vi "GET_Available_TTL_outputs_array.vi"(4 "IO parameters cluster":T1) -> (0 "Disabled items":i32[](array[numeric]), 1 "Available TTL outputs array":cluster{"String":string, "Value":i32}[](array[cluster]))   [LabVIEW 2018, in "Tracker.lvlib"]
uses:
  Tracker.lvlib
  Controls/CTL_IO_params_cluster.ctl
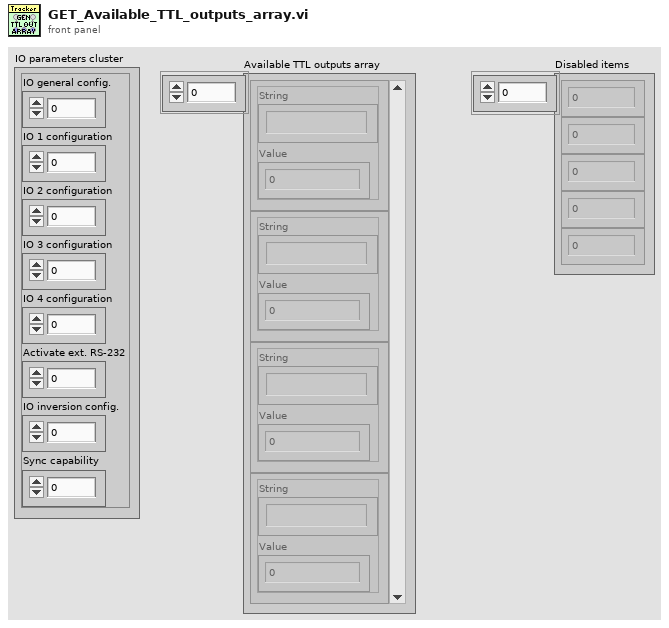
[diagram p1: front panel]
types:
  T1 = typedef "Tracker.lvlib/CTL_IO_params_cluster.ctl" = cluster{"IO general config.":u16, "IO 1 configuration":u16, "IO 2 configuration":u16, "IO 3 configuration":u16, "IO 4 configuration":u16, "Activate ext. RS-232":u16, "IO inversion config.":u16, "Sync capability":u8}
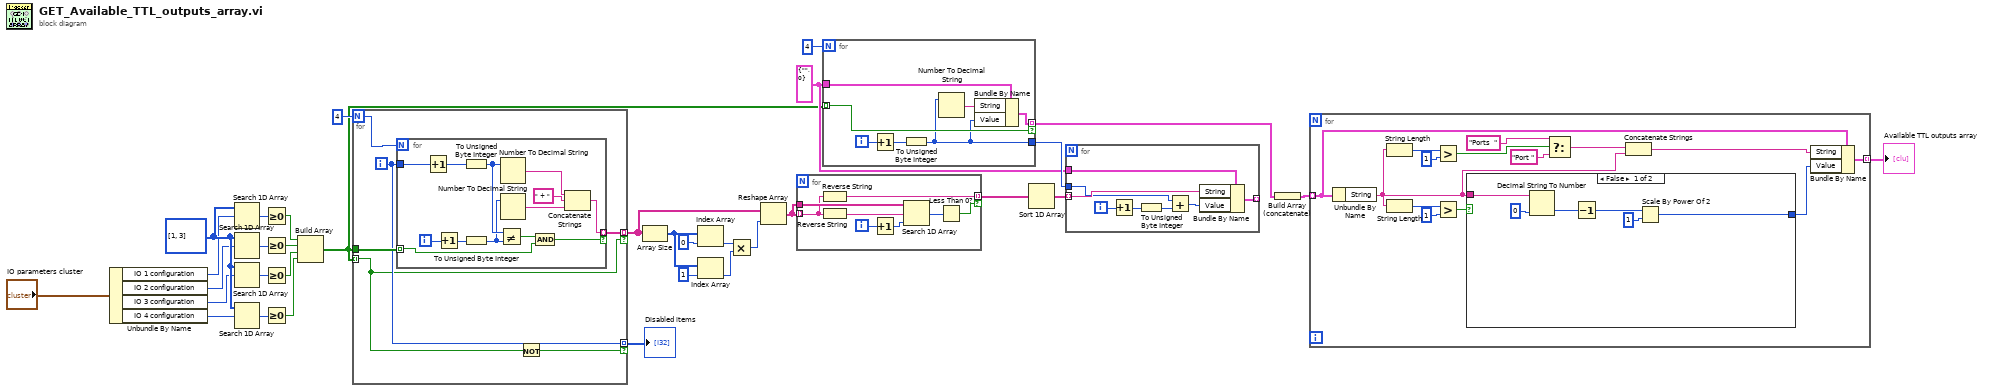
[diagram p0: block diagram]
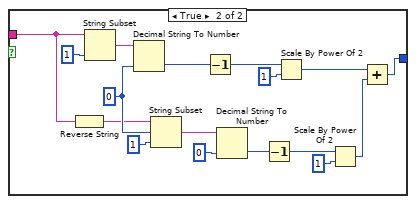
[diagram p2: hidden frame]
diagram:
  w16 = u16[] [1, 3]
  w22 = cluster{"String":string, "Value":u8} {"String"="", "Value"=0} ("Stim. cluster")
  n1 = Unbundle By Name("IO parameters cluster") -> ("IO 1 configuration"=w15:u16, "IO 2 configuration"=w14:u16, "IO 3 configuration"=w13:u16, "IO 4 configuration"=w12:u16)
  n2 = Search 1D Array(1D array=w16, element=w15) -> (index of element=w11:i32)  [unwired: 1 in]
  n3 = Search 1D Array(1D array=w16, element=w14) -> (index of element=w10:i32)  [unwired: 1 in]
  n4 = Search 1D Array(1D array=w16, element=w13) -> (index of element=w9:i32)  [unwired: 1 in]
  n5 = Search 1D Array(1D array=w16, element=w12) -> (index of element=w8:i32)  [unwired: 1 in]
  n6 = Greater Or Equal To 0?(x=w11) -> (x >= 0?=w7:bool)
  n7 = Greater Or Equal To 0?(x=w10) -> (x >= 0?=w6:bool)
  n8 = Greater Or Equal To 0?(x=w9) -> (x >= 0?=w5:bool)
  n9 = Greater Or Equal To 0?(x=w8) -> (x >= 0?=w4:bool)
  n10 = Build Array(w7, w6, w5, w4) -> (w3:bool[])
  n11 = for {
    N: 4 -> [w39]
    tunnel: [w38] -> w31 mode=indexing if=w35
    tunnel: w3 -> [w35] mode=indexing
    tunnel: w3 -> [w37]
    tunnel: [w36] -> w1 mode=indexing if=w34
    i -> [w36]
    n12 = for {
      N: w39 -> [_]
      tunnel: w36 -> [w51]
      tunnel: [w45] -> w38 mode=indexing if=w41
      tunnel: w37 -> [w40] mode=indexing
      i -> [w52]
      n13 = Increment(x=w51) -> (x+1=w50:i32)
      n14 = Increment(x=w52) -> (x+1=w49:i32)
      n15 = To Unsigned Byte Integer(number=w50) -> (unsigned 8bit integer=w44:u8)
      n16 = To Unsigned Byte Integer(number=w49) -> (unsigned 8bit integer=w43:u8)
      n17 = Not Equal?(x=w44, y=w43) -> (x != y?=w42:bool)
      n18 = Number To Decimal String(number=w44) -> (decimal integer string=w48:string)  [unwired: 1 in]
      n19 = Number To Decimal String(number=w43) -> (decimal integer string=w47:string)  [unwired: 1 in]
      n20 = And(x=w42, y=w40) -> (x .and. y?=w41:bool)
      n21 = Concatenate Strings(w48, " + " ("string"), w47) -> (w45:string)
    }
    n22 = Not(x=w35) -> (.not. x?=w34:bool)
  }
  "Disabled items" <- w1
  n23 = Array Size(array=w31) -> (size(s)=w30:i32[])
  n24 = Index Array(array=w30, index=0) -> (element=w27:i32)
  n25 = Index Array(array=w30, index=1) -> (element=w26:i32)
  n26 = Multiply(x=w27, y=w26) -> (x*y=w25:i32)
  n27 = Reshape Array(w31, w25) -> (w24:string[])
  n28 = for {
    tunnel: w24 -> [w58] mode=indexing
    tunnel: [w53] -> w21 mode=indexing if=w56
    tunnel: w24 -> [w60]
    i -> [w55]
    n29 = Reverse String(1:w58) -> (0:w53:string)
    n30 = Reverse String(1:w58) -> (0:w59:string)
    n31 = Increment(x=w55) -> (x+1=w54:i32)
    n32 = Search 1D Array(1D array=w60, element=w59, start index (0)=w54) -> (index of element=w57:i32)
    n33 = Less Than 0?(x=w57) -> (x < 0?=w56:bool)
  }
  n34 = for {
    N: 4 -> [_]
    tunnel: w3 -> [w62] mode=indexing
    tunnel: w22 -> [w65]
    tunnel: [w63] -> w2 mode=indexing if=w62
    tunnel: [w61] -> w23
    i -> [w67]
    n35 = Increment(x=w67) -> (x+1=w66:i32)
    n36 = To Unsigned Byte Integer(number=w66) -> (unsigned 8bit integer=w61:u8)
    n37 = Number To Decimal String(number=w61) -> (decimal integer string=w64:string)  [unwired: 1 in]
    n38 = Bundle By Name(cluster=w65, "String"=w64, "Value"=w61) -> (w63:cluster{"String":string, "Value":u8})
  }
  n39 = Sort 1D Array(array=w21) -> (sorted array=w20:string[])
  n40 = for {
    tunnel: w20 -> [w73] mode=indexing
    tunnel: w23 -> [w72]
    tunnel: w22 -> [w74]
    tunnel: [w68] -> _ mode=indexing
    i -> [w75]
    n41 = Increment(x=w75) -> (x+1=w71:i32)
    n42 = To Unsigned Byte Integer(number=w71) -> (unsigned 8bit integer=w69:u8)
    n43 = Add(x=w72, y=w69) -> (x+y=w70:u8)
    n44 = Bundle By Name(cluster=w74, "String"=w73, "Value"=w70) -> (w68:cluster{"String":string, "Value":u8})
  }
  n45 = Build Array (concatenate)(w2) -> (w19:cluster{"String":string, "Value":u8}[])
  n46 = for {
    tunnel: w19 -> [w86] mode=indexing
    tunnel: [w85] -> w18 mode=indexing
    n47 = Unbundle By Name(w86) -> ("String"=w79:string)
    n48 = String Length(string=w79) -> (length=w78:i32)
    n49 = String Length(string=w79) -> (length=w89:i32)
    n50 = Greater?(x=w78, y=1) -> (0:w76:bool)
    n51 = Greater?(x=w89, y=1) -> (0:w87:bool)
    n52 = case shown="False" w87 {
      tunnel: w79 -> [w95 w106]
      tunnel: [w90 w96] -> w84
      frame False {
        n53 = Decimal String To Number(string=w95, default (0L)=u8 0 ("default (0 I32)")) -> (number=w91:u8)  [unwired: 1 in, 1 out]
        n54 = Decrement(x=w91) -> (x-1=w92:u8)
        n55 = Scale By Power Of 2(n=w92, x=u8 1) -> (x*2^n=w90:u8)
      }
      frame True {
        w107 = u8 0 ("default (0 I32)")
        n56 = Reverse String(1:w106) -> (0:w105:string)
        n57 = String Subset(string=w106, length (rest)=1 ("length (rest)")) -> (substring=w111:string)  [unwired: 1 in]
        n58 = Decimal String To Number(string=w111, default (0L)=w107) -> (number=w104:u8)  [unwired: 1 in, 1 out]
        n59 = String Subset(string=w105, offset (0)=w107, length (rest)=1 ("length (rest)")) -> (substring=w109:string)
        n60 = Decrement(x=w104) -> (x-1=w103:u8)
        n61 = Decimal String To Number(string=w109, default (0L)=u8 0 ("default (0 I32)")) -> (number=w99:u8)  [unwired: 1 in, 1 out]
        n62 = Decrement(x=w99) -> (x-1=w100:u8)
        n63 = Scale By Power Of 2(n=w103, x=u8 1) -> (x*2^n=w98:u8)
        n64 = Scale By Power Of 2(n=w100, x=u8 1) -> (x*2^n=w97:u8)
        n65 = Add(x=w98, y=w97) -> (x+y=w96:u8)
      }
    }
    n66 = Select(t="Ports  " ("string"), s=w76, f="Port ") -> (s? t:f=w82:string)
    n67 = Concatenate Strings(w82, w79) -> (w83:string)
    n68 = Bundle By Name(cluster=w86, "String"=w83, "Value"=w84) -> (w85:cluster{"String":string, "Value":u8})
  }
  "Available TTL outputs array" <- w18
